vi "Initialize Settings.vi"(7 "error in (no error)":errorcluster, 10 "OD600 in":refnum<class "OD600.lvclass">) -> (0 "error out":errorcluster, 1 "Sampling Interval 2":i32, 2 "VISA out":refnum<visa-resource-name>, 3 "OD600 out":refnum<class "OD600.lvclass">)   [LabVIEW 2013, in "OD600.lvlib" / "OD600.lvclass"]
uses:
  OD600.lvclass
  PluginInterface/PluginInterface.lvlibp/PluginInterfaceClass/Read Name.vi
panel:
  in  "Button":bool
  in  "VISA in":refnum<visa-resource-name>
  in  "Sampling Interval":i32
  in  "String":string
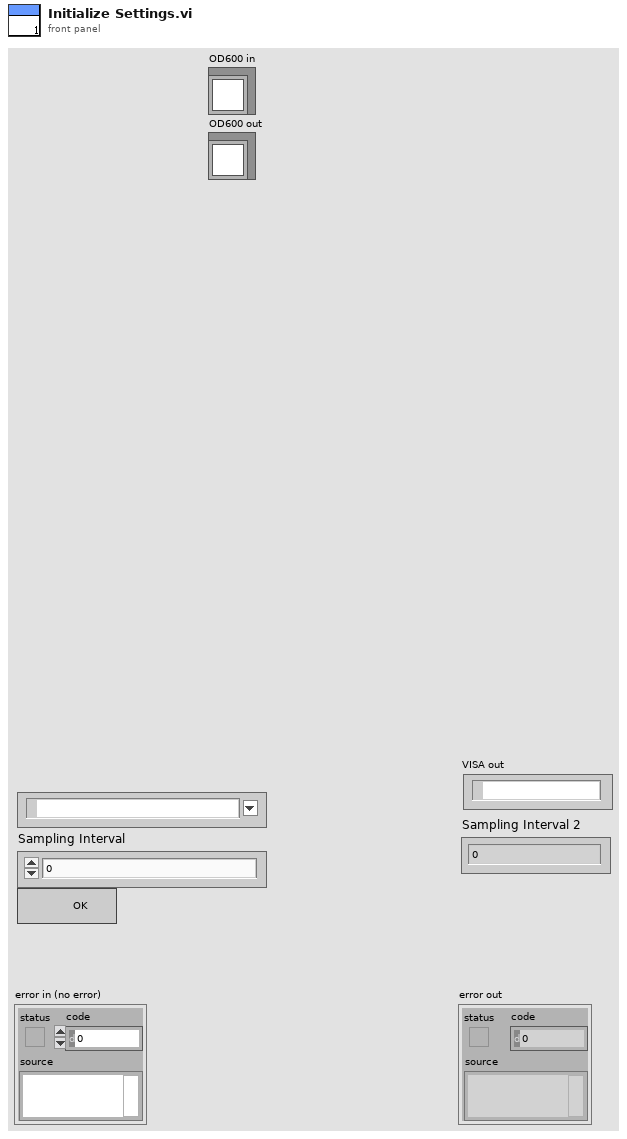
[diagram p1: front panel]
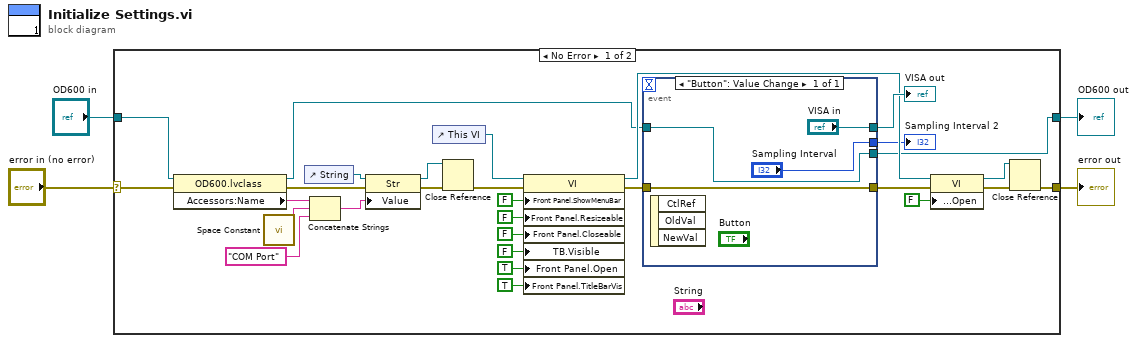
[diagram p0: block diagram]
diagram:
  n1 = case shown="No Error" "error in (no error)" {
    selector: "error in (no error)" -> [w8 w39]
    tunnel: [w19 w39] -> w3
    tunnel: [w18 w38] -> w2
    tunnel: "OD600 in" -> [w9 w38]
    frame No Error {
      n2 = property class="OD600.lvclass"(reference=w9, error in=w8) -> (reference out=w7:refnum<class "OD600.lvclass">, error out=w6:errorcluster, "Accessors:Name"=w5:string)
      n3 = call <vilib>:"Space Constant.vi"() -> ("String"=w10:string)
      n4 = control-ref of="String"() -> (w14:refnum<vi>)
      n5 = Concatenate Strings(w5, w10, "COM Port" ("string")) -> (w17:string)
      n6 = property class="Str"(reference=w14, error in=w6, "Value"=w17) -> (reference out=w16:refnum<vi>, error out=w15:errorcluster)
      n7 = control-ref of="This VI"() -> (w32:refnum<vi>)
      n8 = Close Reference(reference=w16, error in (no error)=w15) -> (error out=w13:errorcluster)
      n9 = property class="VI"(reference=w32, error in=w13, "Front Panel.ShowMenuBar"=FALSE ("Front Panel Window:Show Menu Bar"), "Front Panel.Resizeable"=FALSE ("Front Panel Window:Resizable"), "Front Panel.Closeable"=FALSE ("Front Panel Window:Closeable"), "TB.Visible"=FALSE ("Tool Bar:Visible"), "Front Panel.Open"=TRUE ("Front Panel Window:Open"), "Front Panel.TitleBarVis"=TRUE ("Front Panel Window:Title Bar Visible")) -> (reference out=w21:refnum<vi>, error out=w25:errorcluster)
      n10 = event shown="[0] \"Button\": Value Change" {
        selector: _ -> [_]
        dyn-events: _ -> [_]
        timeout: _ -> [_]
        tunnel: w25 -> [w36]
        tunnel: [w36] -> w20
        tunnel: ["VISA in"] -> w33
        tunnel: w7 -> [w35]
        tunnel: [w35] -> w18
        tunnel: ["Sampling Interval"] -> w12
        event "Button": Value Change {
          n11 = event-data() -> ()  [unwired: 1 in, 3 out]
        }
      }
      "VISA out" <- w33
      "Sampling Interval 2" <- w12
      n12 = property class="VI"(reference=w21, error in=w20, "Front Panel.Open"=FALSE ("Front Panel Window:Open")) -> (reference out=w24:refnum<vi>, error out=w23:errorcluster)
      n13 = Close Reference(reference=w24, error in (no error)=w23) -> (error out=w19:errorcluster)
    }
    frame Error {
    }
  }
  "error out" <- w3
  "OD600 out" <- w2
